vi "NI VeriStand - Write Multiple Waveforms (CDB).vi"(8 "error in (no error)":errorcluster, 9 "timeout in ms (0)":i32, 10 "Data":cdb[][](array[numeric]), 11 "Multiple Waveforms Write Session (CDB) in":refnum<class "Multiple Waveforms Write (CDB).lvclass">) -> (0 "error out":errorcluster, 1 "timed out?":bool, 3 "Multiple Waveforms Write Session (CDB) out":refnum<class "Multiple Waveforms Write (CDB).lvclass">)   [LabVIEW 2020, in "NI_VS Custom Device Waveform API.lvlib" / "Multiple Waveforms Write (CDB).lvclass"]
doc: "Writes an array of values to the waveform(s) associated with the specified write session. Use the Start Waveform(s) VI prior to this VI to set the waveform start time (t0) or start times. NI VeriStand considers all data this VI writes to be continuous unless the Start Waveform(s) VI executes again with a different start time."
uses:
  Multiple Waveforms Write (CDB).lvclass
  D:/p4/penguin/lvaddon/Veristand/master/src/LabVIEW/vilib/NI VeriStand/Custom Device Waveform API/Waveform Session.lvclass
  Waveform Session.lvclass/Waveform Session.ctl
  Multiple Waveforms Write (CDB).lvclass/Multiple Waveforms Write (CDB).ctl
  Internal Comm Classes/WPL Comm/WPL Comm (2D CDB)/WPL Comm (2D CDB).lvclass/WPL Comm (2D CDB).ctl
  Internal Comm Classes/WPL Comm/WPL Comm.lvclass/WPL Comm.ctl
  Internal Comm Classes/WPL Comm/Direct Send WPL Command.vi
  Internal Comm Classes/WPL Comm/Convert Q Error to Shutdown Error.vi
  Internal Comm Classes/WPL Comm/WPL Comm (2D CDB)/WPL Comm (2D CDB).lvclass
  D:/p4/penguin/lvaddon/Veristand/master/src/LabVIEW/vilib/NI VeriStand/Custom Device Waveform API/Internal Comm Classes/WPL Comm/WPL Comm.lvclass
  <vilib>/Utility/error.llb/Error Cluster From Error Code.vi
  Waveform Session.lvclass
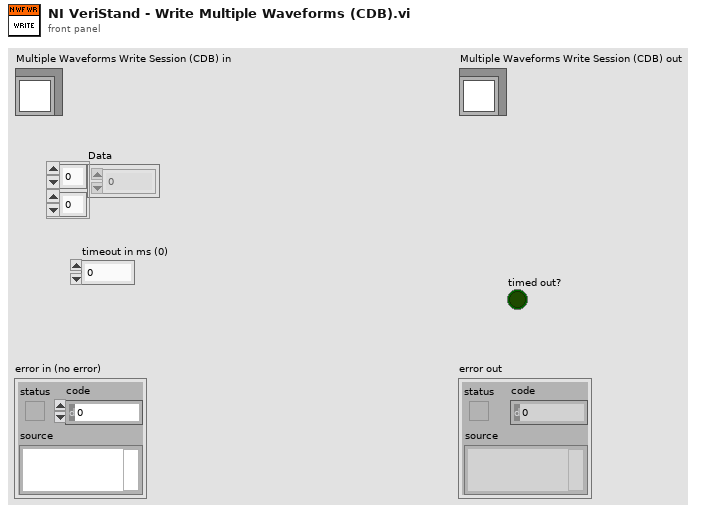
[diagram p1: front panel]
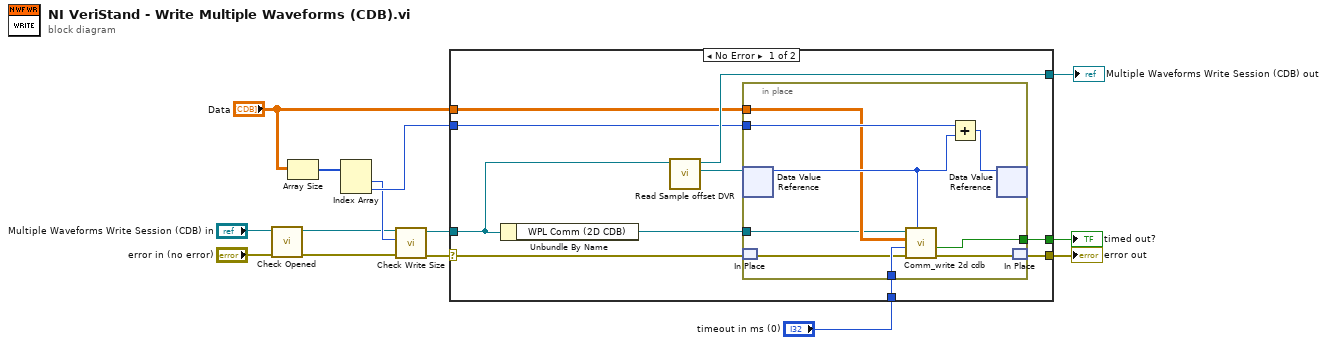
[diagram p0: block diagram]
diagram:
  n1 = call "Check Opened.vi"("error in (no error)"="error in (no error)", "Waveform Session in"="Multiple Waveforms Write Session (CDB) in") -> ("error out"=w2:errorcluster, "Waveform Session out"=w1:refnum<class "Multiple Waveforms Write (CDB).lvclass">)  [unwired: 8 in]
  n2 = Array Size(array="Data") -> (size(s)=w6:i32[])
  n3 = Index Array(array=w6) -> (element #1=w5:i32, element #2=w8:i32)  [unwired: 2 in]
  n4 = call "Check Write Size.vi"("error in (no error)"=w2, "# Of Waveforms"=w5, "Waveform Session in"=w1) -> ("error out"=w10:errorcluster, "Waveform Session out"=w9:refnum<class "Multiple Waveforms Write (CDB).lvclass">)  [unwired: 7 in]
  n5 = case shown="No Error" w10 {
    selector: w10 -> [w20 w35]
    tunnel: [w24 w35] -> w14
    tunnel: [w21 w34] -> w13
    tunnel: "Data" -> [w18 _]
    tunnel: [w23 _] -> w12
    tunnel: "timeout in ms (0)" -> [w22 _]
    tunnel: w9 -> [w16 w34]
    tunnel: w8 -> [w19 _]
    frame No Error {
      n6 = Unbundle By Name(w16) -> ("WPL Comm (2D CDB)"=w15:refnum<class "WPL Comm (2D CDB).lvclass">)
      n7 = call "Read Sample offset DVR.vi"("Waveform Session in"=w16) -> ("Sample offset"=w17:refnum<data-value>, "Waveform Session out"=w21:refnum<class "Multiple Waveforms Write (CDB).lvclass">)  [unwired: 9 in]
      n8 = in-place {
        in-place-border: [w32] -> w23
        in-place-border: w22 -> [w31]
        in-place-border: w19 -> [w30]
        in-place-border: w18 -> [w28]
        in-place-border: w15 -> [w26]
        n9 = in-place-dvr #1(w17) -> (w29:u64)  [unwired: 1 out]
        n10 = in-place-match #2(w20) -> (w25:errorcluster)
        n11 = call "Comm_write 2d cdb.vi"("Sample Offset"=w29, "error in (no error)"=w25, "timeout in ms (0)"=w31, "Data"=w28, "WPL Comm (2D CDB) in"=w26) -> ("error out"=w27:errorcluster, "timed out?"=w32:bool)  [unwired: 4 in, 1 out]
        n12 = Add(x=w30, y=w29) -> (x+y=w33:u64)
        n13 = in-place-dvr #1(w33) -> ()  [unwired: 2 out]
        n14 = in-place-match #2(w27) -> (w24:errorcluster)
      }
    }
    frame Error {
    }
  }
  "error out" <- w14
  "Multiple Waveforms Write Session (CDB) out" <- w13
  "timed out?" <- w12
